vi "Scan Initilize_without Accurate Measure_ver2.vi"(8 "error in (no error)":errorcluster, 9 "Current Setting":u8[](array[numeric]), 10 "Channel Count":i32, 11 "VISA Refnum in":refnum<visa-resource-name>) -> (0 "error out":errorcluster, 1 "N channel number":i32, 2 "P channel number":i32, 3 "VISA Refnum out":refnum<visa-resource-name>, 5 "Current Channel":string[](array[string]))   [LabVIEW 2023]
uses:
  <instrlib>/Agilent 3446X Series/Agilent 3446X Series.lvlib
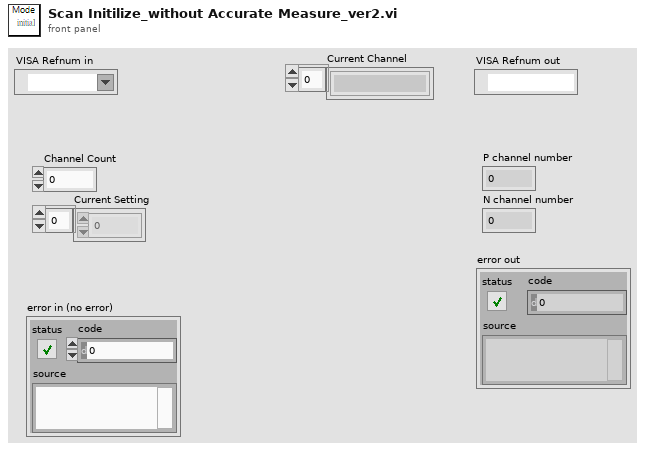
[diagram p1: front panel]
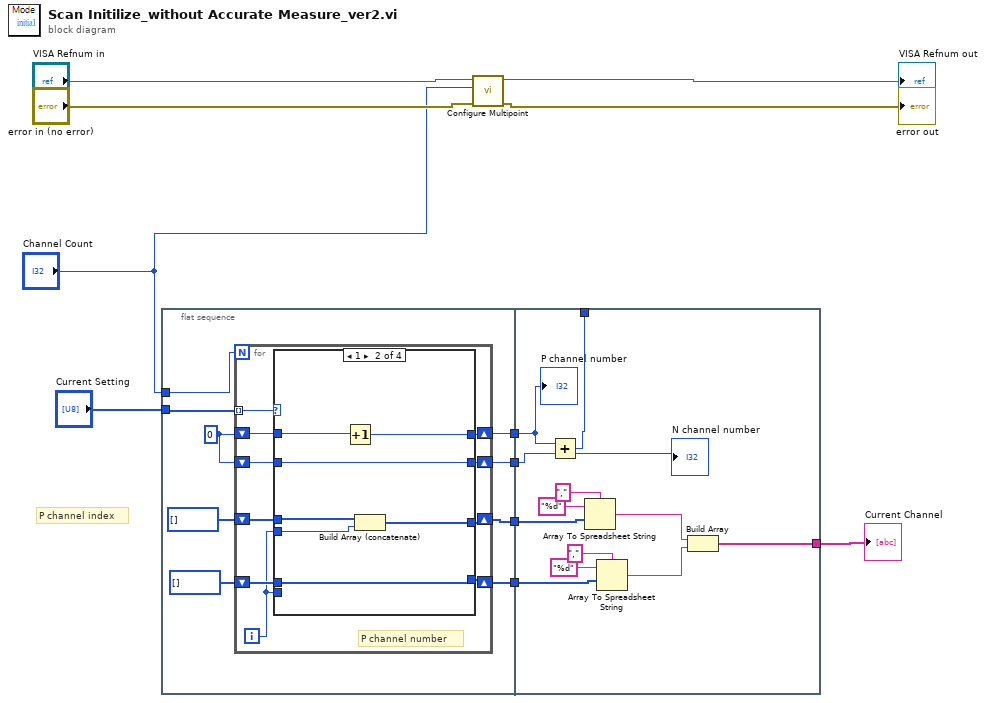
[diagram p0: block diagram]
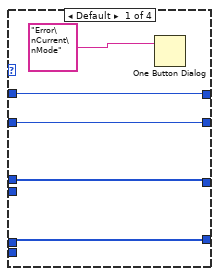
[diagram p2: hidden frame]
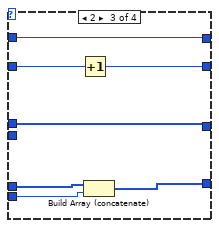
[diagram p3: hidden frame]
diagram:
  # "P channel index"
  # "P channel number"
  n1 = flat-sequence {
    tunnel: "Channel Count" -> [w20]
    tunnel: "Current Setting" -> [w19]
    tunnel: [w17] -> w7
    tunnel: [w16] -> w6
    tunnel: [w13] -> w5
    tunnel: [w12] -> w4
    tunnel: w7 -> [w65]
    tunnel: w6 -> [w64]
    tunnel: [w63] -> _
    tunnel: w5 -> [w60]
    tunnel: w4 -> [w57]
    tunnel: [w54] -> w2
    frame #0 {
      w18 = 0 ("P_current_count")
      n2 = for {
        N: w20 -> [_]
        tunnel: w19 -> [w30] mode=indexing
        shift-right: [w28] -> w17
        shift-left: w18 -> [w29]
        shift-right: [w26] -> w16
        shift-left: w18 -> [w27]
        shift-right: [w24] -> w13
        shift-left: i32[] [] -> [w25]
        shift-right: [w22] -> w12
        shift-left: i32[] [] -> [w23]
        i -> [w21]
        n3 = case shown="1" w30 {
          tunnel: w29 -> [w34 w42 w47 w53]
          tunnel: [w34 w41 w47 w53] -> w28
          tunnel: w27 -> [w33 w40 w49 w52]
          tunnel: [w33 w40 w48 w52] -> w26
          tunnel: w25 -> [w31 w39 w43 w51]
          tunnel: w21 -> [_ w38 _ _]
          tunnel: [w31 w37 w43 w51] -> w24
          tunnel: w23 -> [w32 w36 w46 w50]
          tunnel: [w32 w36 w45 w50] -> w22
          tunnel: w21 -> [_ _ w44 _]
          frame Default {
            n4 = One Button Dialog(message="Error\nCurrent\nMode" ("error source (\" \")")) -> ()  [unwired: 1 in, 1 out]
          }
          frame 1 {
            n5 = Increment(x=w42) -> (x+1=w41:i32)
            n6 = Build Array (concatenate)(w39, w38) -> (w37:i32[])
          }
          frame 2 {
            n7 = Increment(x=w49) -> (x+1=w48:i32)
            n8 = Build Array (concatenate)(w46, w44) -> (w45:i32[])
          }
          frame 0 {
          }
        }
      }
    }
    frame #1 {
      n9 = Add(x=w65, y=w64) -> (x+y=w63:i32)
      n10 = Array To Spreadsheet String(delimiter (Tab)=",", array=w60, 3:"%d" ("format string")) -> (spreadsheet string=w56:string)
      n11 = Array To Spreadsheet String(delimiter (Tab)=",", array=w57, 3:"%d" ("format string")) -> (spreadsheet string=w55:string)
      n12 = Build Array(w56, w55) -> (w54:string[])
      "P channel number" <- w65
      "N channel number" <- w64
    }
  }
  n13 = call <instrlib>:"Configure Multipoint.vi"("error in (no error)"="error in (no error)", "Trigger Count (1)"="Channel Count", "VISA resource name"="VISA Refnum in") -> ("error out"=→"error out":errorcluster, "VISA resource name out"=→"VISA Refnum out":refnum<visa-resource-name>)  [unwired: 4 in, 3 out]
  "Current Channel" <- w2
